vi "Get Inst Power Setting.vi"(8 "error in (no error)":errorcluster, 11 "niDTS BT DUT in":refnum<class "niDTS BT Dut.lvclass">) -> (0 "error out":errorcluster, 2 "Instrument Power":dbl, 3 "niDTS BT DUT out":refnum<class "niDTS BT Dut.lvclass">)   [LabVIEW 2015, in "niDTS BT.lvlib" / "niDTS BT Dut.lvclass"]
uses:
  niDTS BT Dut.lvclass
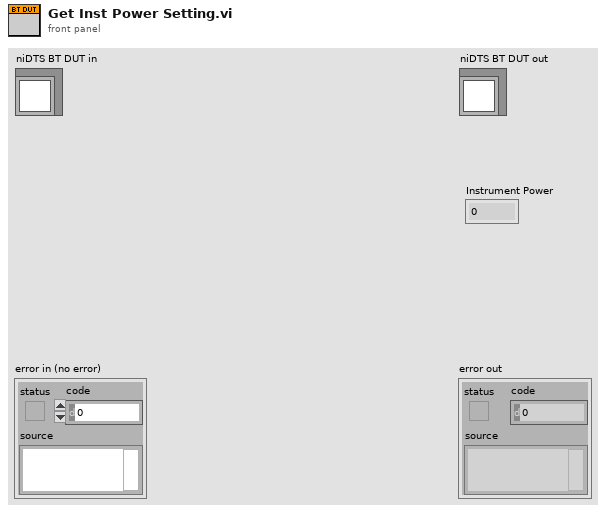
[diagram p1: front panel]
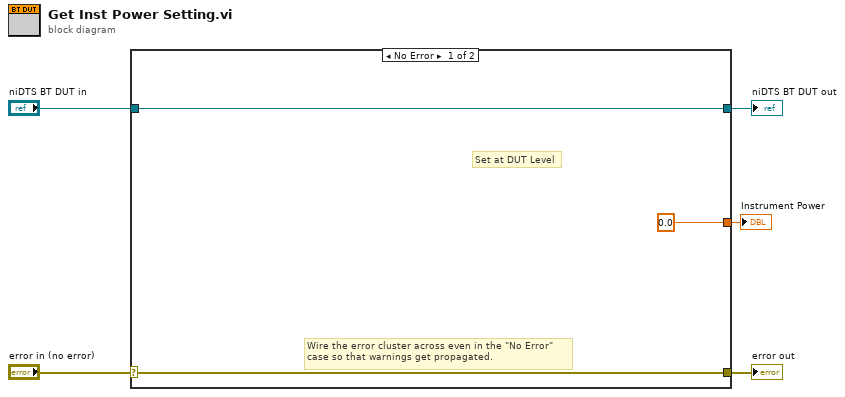
[diagram p0: block diagram]
diagram:
  n1 = case shown="No Error" "error in (no error)" {
    selector: "error in (no error)" -> [w7 w10]
    tunnel: [w7 w10] -> w4
    tunnel: [w8 w9] -> w2
    tunnel: "niDTS BT DUT in" -> [w8 w9]
    tunnel: [0.0 _] -> w1
    frame No Error {
      # "Set at DUT Level"
      # "Wire the error cluster across even in the \"No Error\"\ncase so that warnings get propagated."
    }
    frame Error {
    }
  }
  "error out" <- w4
  "niDTS BT DUT out" <- w2
  "Instrument Power" <- w1
